vi "WMI Set Brightness.vi"() -> ()   [LabVIEW 2012]
doc: "Set the monitor brightness using the Windows Management Instrumentation infrastructure. The scale of brightness is an integer ranging in value from 0-100.\n\n© 2014 MSR Consulting, LLC. All rights reserved."
uses:
  System.Management
panel:
  in  "Brightness":i8(slide)=100 min=0 max=100 scale=0.0..100.0
  out "error out":errorcluster
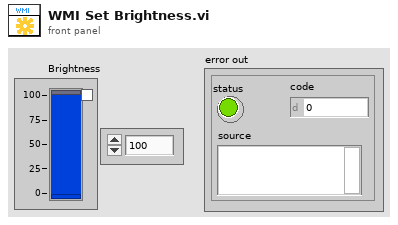
[diagram p1: front panel]
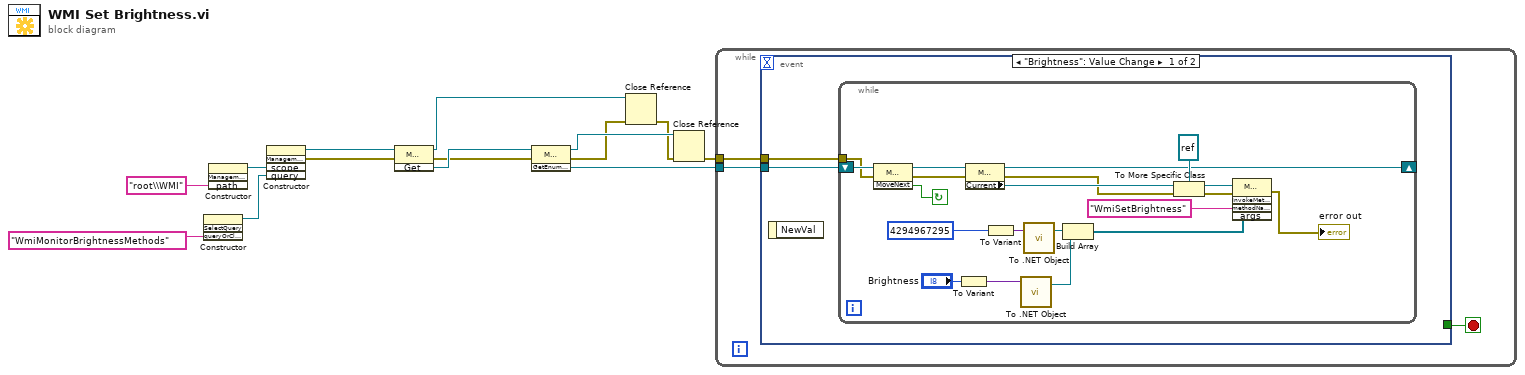
[diagram p0: block diagram]
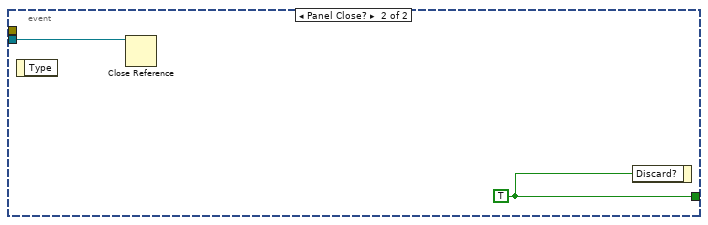
[diagram p2: hidden frame]
diagram:
  n1 = constructor class="SelectQuery"("queryOrClassName"="WmiMonitorBrightnessMethods") -> (reference out=w6:refnum<k24>)  [unwired: 3 in, 3 out]
  n2 = constructor class="ManagementScope"("path"="root\\WMI") -> (reference out=w8:refnum<k24>)  [unwired: 3 in, 3 out]
  n3 = constructor class="ManagementObjectSearcher"("scope"=w8, "query"=w6) -> (reference out=w14:refnum<k24>, error out=w11:errorcluster)  [unwired: 3 in, 3 out]
  n4 = invoke class="ManagementObjectSearcher" method="Get"(reference=w14, error in=w11) -> (reference out=w5:refnum<k24>, error out=w10:errorcluster, "Get"=w13:refnum<k24>)  [unwired: 1 in]
  n5 = invoke class="ManagementObjectCollection" method="GetEnumerator"(reference=w13, error in=w10) -> (reference out=w4:refnum<k24>, error out=w3:errorcluster, "GetEnumerator"=w12:refnum<k24>)  [unwired: 1 in]
  n6 = Close Reference(reference=w5, error in (no error)=w3) -> (error out=w2:errorcluster)
  n7 = Close Reference(reference=w4, error in (no error)=w2) -> (error out=w1:errorcluster)
  n8 = while {
    tunnel: w1 -> [w17]
    tunnel: w12 -> [w16]
    stop <- w15 stop-if-true
    n9 = event shown="[0] \"Brightness\": Value Change" {
      selector: _ -> [_ _]
      dyn-events: _ -> [_ _]
      timeout: _ -> [_ _]
      tunnel: w17 -> [w19 _]
      tunnel: w16 -> [w18 w40]
      tunnel: [_ w41] -> w15
      event "Brightness": Value Change {
        n10 = event-data() -> ()  [unwired: 1 in, 1 out]
        n11 = while {
          shift-right: [w30] -> _
          shift-left: w18 -> [w39]
          tunnel: w19 -> [w35]
          stop <- w38 continue-if-true
          n12 = invoke class="ManagementObjectCollection+Mana" method="MoveNext"(reference=w39, error in=w35) -> (reference out=w37:refnum<k24>, error out=w36:errorcluster, "MoveNext"=w38:bool)  [unwired: 1 in]
          n13 = To Variant(anything="Brightness") -> (Variant=w28:variant)
          n14 = property class="ManagementObjectCollection+Mana"(reference=w37, error in=w36) -> (reference out=w30:refnum<k24>, error out=w22:errorcluster, "Current"=w34:refnum<k24>)
          n15 = To Variant(anything=u32 4294967295) -> (Variant=w29:variant)
          n16 = call <vilib>:"To .NET Object.vi"("anything"=w28) -> (".NET object"=w25:refnum<k24>)  [unwired: 1 in, 1 out]
          n17 = call <vilib>:"To .NET Object.vi"("anything"=w29) -> (".NET object"=w26:refnum<k24>)  [unwired: 1 in, 1 out]
          n18 = Build Array(w26, w25) -> (w24:refnum<k24>[])
          n19 = To More Specific Class(target class=refnum<k24> refnum ("Current"), reference=w34, error in=w22) -> (specific class reference=w32:refnum<k24>, error out=w21:errorcluster)
          n20 = invoke class="ManagementObject" method="InvokeMethod"(reference=w32, error in=w21, "methodName"="WmiSetBrightness", "args"=w24) -> (error out=→"error out":errorcluster)  [unwired: 1 in, 4 out]
        }
      }
      event Panel Close? {
        w41 = TRUE
        n21 = event-data() -> ()  [unwired: 1 in, 1 out]
        n22 = Close Reference(reference=w40) -> ()  [unwired: 1 in, 1 out]
        n23 = event-data("Discard?"=w41) -> ()  [unwired: 1 in, 1 out]
      }
    }
  }
